vi "RSZVB Set Pulse Section Limit Lines State.vi"(4 "Record Number (1)":i32=1, 5 "Limit Lines State (F: Off)":bool, 6 "Generator/Port Number (1)":i32=1, 7 "Interface Type (0: Generator)":i32(ring) items=["Generator", "Analyzer Source"], 8 "error in (no error)":errorcluster {"code" format="%.0x"}, 9 "Receiver Type (0: A)":i32(ring) items=["A", "B"], 10 "Channel (1)":i32=1, 11 "VISA session":refnum<visa-resource-name>) -> (0 "error out":errorcluster {"code" format="%.0x"}, 3 "dup VISA session":refnum<visa-resource-name>)   [LabVIEW 2011]
doc: "This VI displays or hides the limit lines of the averaging section for the wave quantity. \n\nRemote-control command(s):\n[SENSe<Ch>:]PULSe:RECeiver:A<rec_no>:GENerator<gen_no>:LINEs[:STATe] <Boolean>\n[SENSe<Ch>:]PULSe:RECeiver:A<rec_no>:SRCPort<port_no>:LINEs[:STATe] <Boolean>\n[SENSe<Ch>:]PULSe:RECeiver:B<rec_no>:GENerator<gen_no>:LINEs[:STATe] <Boolean>\n[SENSe<Ch>:]PULSe:RECeiver:B<rec_no>:SRCPort<port_no>:LINEs[:STATe] <Boolean>"
uses:
  _utility/RSZVB Global Data.vi
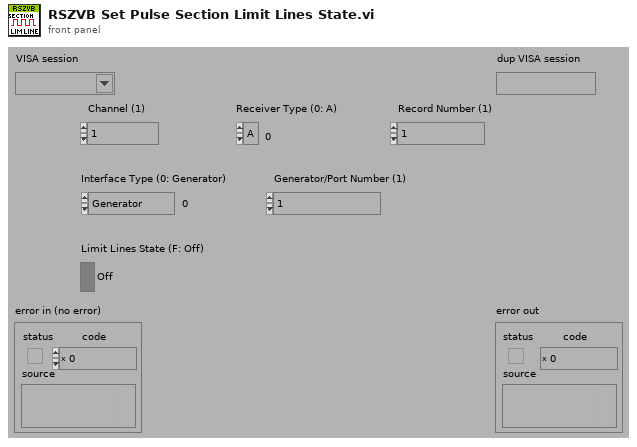
[diagram p1: front panel]
types:
  T1 = cluster{"Error Checking (T: On)":bool, "Installed Options":string[], "Data Valid?":bool, "Ports":i32, "Model":string[], "Option Checking (T: On)":bool}[]
  T2 = cluster{"Error Checking (T: On)":bool, "Installed Options":string[], "Data Valid?":bool, "Ports":i32, "Model":string[], "Option Checking (T: On)":bool}
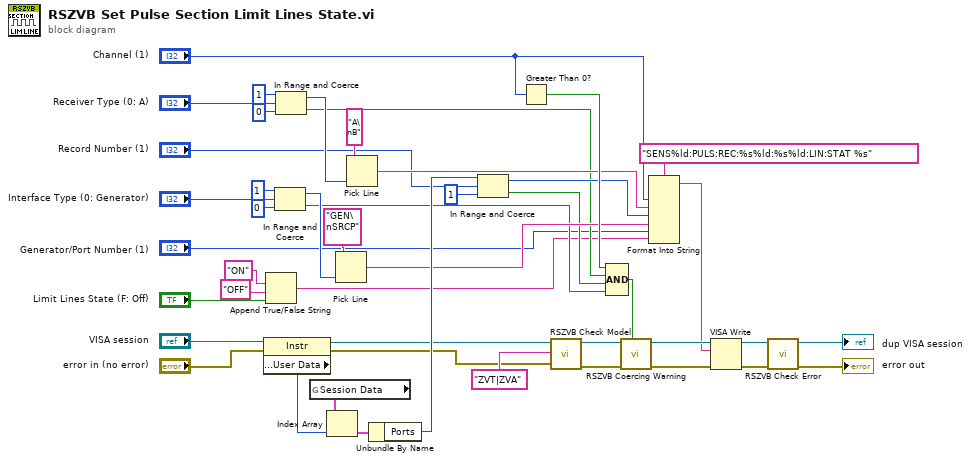
[diagram p0: block diagram]
diagram:
  n1 = property class="Instr"(reference="VISA session", error in="error in (no error)") -> (reference out=w22:refnum<visa-resource-name>, error out=w21:errorcluster, "General Settings:User Data"=w24:u32)
  n2 = Append True/False String(1:"Limit Lines State (F: Off)", 2:"OFF", 3:"ON") -> (0:w2:string)  [unwired: 1 in]
  n3 = In Range and Coerce(upper limit=1, x="Interface Type (0: Generator)", lower limit=0) -> (coerced(x)=w27:i32, In Range?=w14:bool)
  n4 = In Range and Coerce(upper limit=1, x="Receiver Type (0: A)", lower limit=0) -> (coerced(x)=w31:i32, In Range?=w16:bool)
  n5 = global read "RSZVB Global Data.vi" "Session Data"() -> (w25:T1)
  n6 = Index Array(array=w25, index=w24) -> (element=w26:T2)
  n7 = Pick Line(multi-line string="GEN\nSRCP", line index=w27) -> (output string=w17:string)  [unwired: 1 in]
  n8 = Pick Line(multi-line string="A\nB", line index=w31) -> (output string=w19:string)  [unwired: 1 in]
  n9 = Unbundle By Name(w26) -> ("Ports"=w23:i32)
  n10 = In Range and Coerce(upper limit=w23, x="Record Number (1)", lower limit=1) -> (coerced(x)=w18:i32, In Range?=w15:bool)
  n11 = Greater Than 0?(x="Channel (1)") -> (x > 0?=w38:bool)
  n12 = call "RSZVB Check Model.vi"("error in (no error)"=w21, "Model"="ZVT|ZVA" ("Options"), "VISA session"=w22) -> ("error out"=w36:errorcluster, "dup VISA session"=w35:refnum<visa-resource-name>)  [unwired: 7 in]
  n13 = Compound Arithmetic op=AND(w38, w16, w15, w14) -> (w40:bool)
  n14 = call "RSZVB Coercing Warning.vi"("In Range?"=w40, "error in (no error)"=w36, "VISA session"=w35) -> ("error out"=w43:errorcluster, "dup VISA session"=w44:refnum<visa-resource-name>)  [unwired: 7 in]
  n15 = Format Into String(format string="SENS%ld:PULS:REC:%s%ld:%s%ld:LIN:STAT %s", "Channel (1)", w19, w18, w17, "Generator/Port Number (1)", w2) -> (resulting string=w39:string)  [unwired: 2 in, 1 out]
  n16 = VISA Write(VISA resource name=w44, write buffer=w39, error in (no error)=w43) -> (VISA resource name out=w41:refnum<visa-resource-name>, error out=w42:errorcluster)  [unwired: 1 out]
  n17 = call "RSZVB Check Error.vi"("error in (no error)"=w42, "VISA session"=w41) -> ("error out"=→"error out":errorcluster, "dup VISA session"=→"dup VISA session":refnum<visa-resource-name>)  [unwired: 8 in]
